vi "heater_ctl_wrapper.vi"(4 "Numeric in":i32, 5 "Subtag":string, 6 "String":string, 7 "DataMap":refnum<data-value>, 8 "HeaterTag":string, 9 "DataIndex":i32, 10 "Accessors:CVT Session":T1, 11 "Message Enqueuer in":refnum<class "Message Enqueuer.lvclass">) -> (2 "Numeric out":i32, 3 "Boolean":bool)   [LabVIEW 2017, in "Controller.lvlib" / "gController.lvclass"]
uses:
  gController.lvclass
  <vilib>/ActorFramework/Message Enqueuer/Message Enqueuer.lvclass
  <vilib>/MSR Consulting, LLC/General Reuse/Session APIs/_Session Fwk/Typedefs/Session Handle.ctl
  <vilib>/MSR Consulting, LLC/General Reuse/Session APIs/_Session Fwk/Session - Root.lvclass
  Messages/Update Heater DC MSG/Update Heater DC MSG.lvclass
  C:/Program Files (x86)/National Instruments/LabVIEW 2017/vi.lib/ActorFramework/Message/Message.lvclass
  Data/SOAP Data.lvclass
  Data/SOAP Data.lvclass/SOAP Data.ctl
  <vilib>/ActorFramework/Message Enqueuer/Message Enqueuer.lvclass/Message Enqueuer.ctl
  Data/Read temperatures.vi
  <vilib>/addons/control/pid/pid.llb/PID (DBL).vi
  <vilib>/ActorFramework/Message Priority Queue/Priority Enqueue.vi
  <vilib>/MSR Consulting, LLC/General Reuse/Session APIs/CVT/CVT.lvclass
  <vilib>/addons/control/pid/NI_PID_pid.lvlib
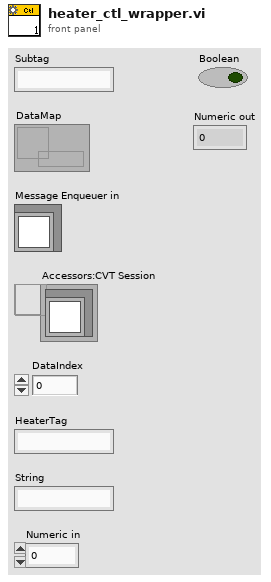
[diagram p1: front panel]
types:
  T1 = typedef "Session - Root.lvclass/Session Handle.ctl" = refnum<data-value>
  T2 = cluster{"pas_cell_1":sgl, "pas_cell_2":sgl, "pas_las_head_1":sgl, "pas_las_head_2":sgl, "cjc0":sgl, "box_exit":sgl, "crd_heater":sgl, "box_inlet":sgl, "crd_laser_head":sgl, "cjc1":sgl}
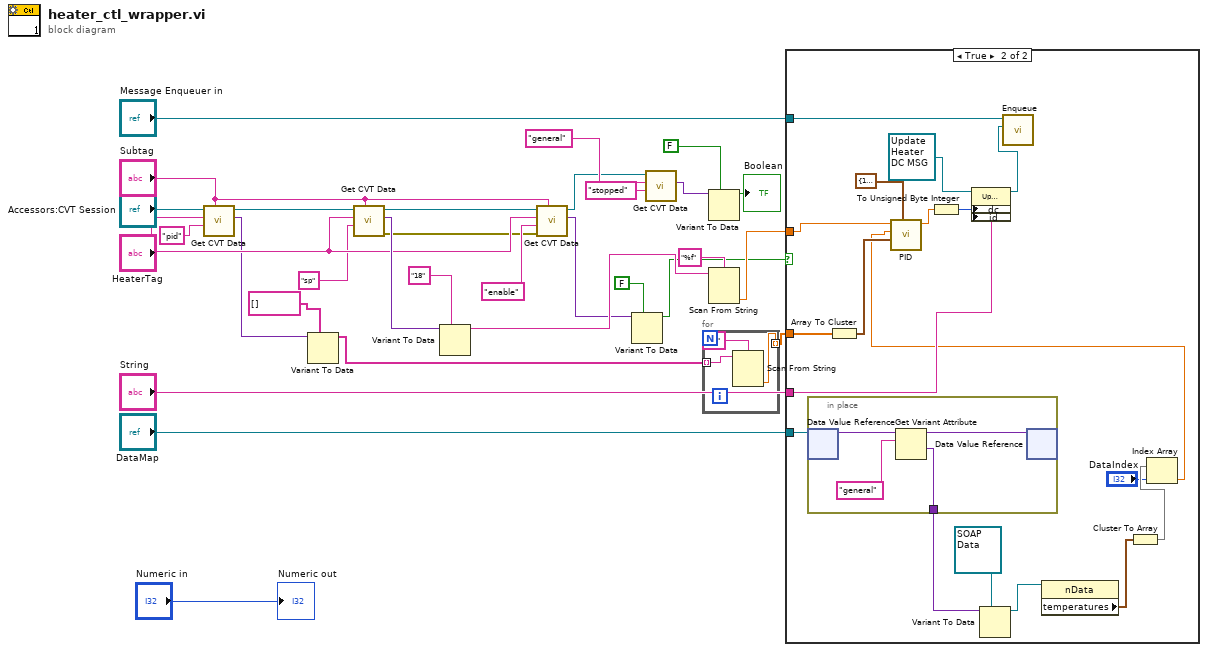
[diagram p0: block diagram]
diagram:
  n1 = call <vilib>:"Get CVT Data.vi"("Subgroup"="Subtag", "Variable"="pid", "Group"="HeaterTag", "CVT Session In"="Accessors:CVT Session") -> ("Data Out"=w5:variant, "CVT Session Out"=w3:T1)  [unwired: 4 in, 2 out]
  n2 = Variant To Data(type=string[] [], Variant=w5) -> (data=w26:string[])  [unwired: 1 in, 1 out]
  n3 = call <vilib>:"Get CVT Data.vi"("Subgroup"="Subtag", "Variable"="sp", "Group"="HeaterTag", "CVT Session In"=w3) -> ("error out"=w7:errorcluster, "Data Out"=w12:variant, "CVT Session Out"=w6:T1)  [unwired: 4 in, 1 out]
  n4 = Variant To Data(type="18", Variant=w12) -> (data=w28:string)  [unwired: 1 in, 1 out]
  n5 = call <vilib>:"Get CVT Data.vi"("Subgroup"="Subtag", "error in"=w7, "Variable"="enable", "Group"="HeaterTag", "CVT Session In"=w6) -> ("Data Out"=w14:variant, "CVT Session Out"=w20:T1)  [unwired: 3 in, 2 out]
  n6 = Variant To Data(type=FALSE, Variant=w14) -> (data=w15:bool)  [unwired: 1 in, 1 out]
  n7 = call <vilib>:"Get CVT Data.vi"("Variable"="stopped", "Group"="general", "CVT Session In"=w20) -> ("Data Out"=w23:variant)  [unwired: 5 in, 3 out]
  n8 = for {
    tunnel: w26 -> [w34] mode=indexing
    tunnel: [w32] -> w27 mode=indexing
    n9 = Scan From String(format string="%f", input string=w34) -> (output 1=w32:dbl)  [unwired: 3 in, 3 out]
  }
  n10 = Variant To Data(type=FALSE, Variant=w23) -> (data=→"Boolean":bool)  [unwired: 1 in, 1 out]
  n11 = Scan From String(format string="%f", input string=w28) -> (output 1=w30:dbl)  [unwired: 3 in, 3 out]
  n12 = case shown="True" w15 {
    tunnel: w27 -> [_ w51]
    tunnel: "Message Enqueuer in" -> [_ w49]
    tunnel: "DataMap" -> [_ w44]
    tunnel: "String" -> [_ w37]
    tunnel: w30 -> [_ w35]
    frame False {
    }
    frame True {
      n13 = in-place {
        in-place-border: [w53] -> w43
        n14 = in-place-dvr #1(w44) -> (w56:variant)  [unwired: 1 out]
        n15 = Get Variant Attribute(Variant=w56, name="general") -> (duplicate Variant=w55:variant, value=w53:variant)  [unwired: 2 in, 2 out]
        n16 = in-place-dvr #1(w55) -> ()  [unwired: 2 out]
      }
      n17 = Array To Cluster(array=w51) -> (cluster=w50:cluster{"[0]":dbl, "[1]":dbl, "[2]":dbl})
      n18 = Variant To Data(type=refnum<class "SOAP Data.lvclass"> refnum ("Controller.lvlib:nData"), Variant=w43) -> (data=w41:refnum<class "SOAP Data.lvclass">)  [unwired: 1 in, 1 out]
      n19 = property class="nData"(reference=w41) -> ("temperatures"=w40:T2)  [unwired: 1 in, 2 out]
      n20 = Cluster To Array(cluster=w40) -> (array=w39:sgl[])
      n21 = Index Array(array=w39, index="DataIndex") -> (element=w36:sgl)
      n22 = call-poly <vilib>:"PID.vi"("output range"=cluster{"output high":dbl, "output low":dbl} {"output high"=100.0, "output low"=0.0}, "PID gains"=w50, "process variable"=w36, "setpoint"=w35) -> ("output"=w47:dbl)  [unwired: 6 in, 1 out]
      n23 = To Unsigned Byte Integer(number=w47) -> (unsigned 8bit integer=w46:u8)
      n24 = property class="Update Heater DC MSG"(reference=refnum<class "Update Heater DC MSG.lvclass"> refnum ("Controller.lvlib:Update Heater DC MSG"), "dc"=w46, "id"=w37) -> (reference out=w45:refnum<class "Update Heater DC MSG.lvclass">)  [unwired: 1 in, 1 out]
      n25 = call <vilib>:"Enqueue.vi"("Message"=w45, "Message Enqueuer in"=w49) -> ()  [unwired: 8 in, 2 out]
    }
  }
  "Numeric out" <- "Numeric in"
